vi "DSF Transfer Group.Separate Rx and Tx.vi"(8 "error in (no error)":errorcluster, 11 "Transfer Groups":refnum<class "Transfer Group.lvclass">[](array[class])) -> (0 "error out":errorcluster, 2 "Tx Transfer Groups":refnum<class "Transfer Group.lvclass">[](array[class]), 3 "Rx Transfer Groups":refnum<class "Transfer Group.lvclass">[](array[class]))   [LabVIEW 2017, in "DSF Core.lvlib" / "Transfer Group.lvclass"]
uses:
  Transfer Group.lvclass
  Transfer Group.lvclass/Transfer Group.ctl
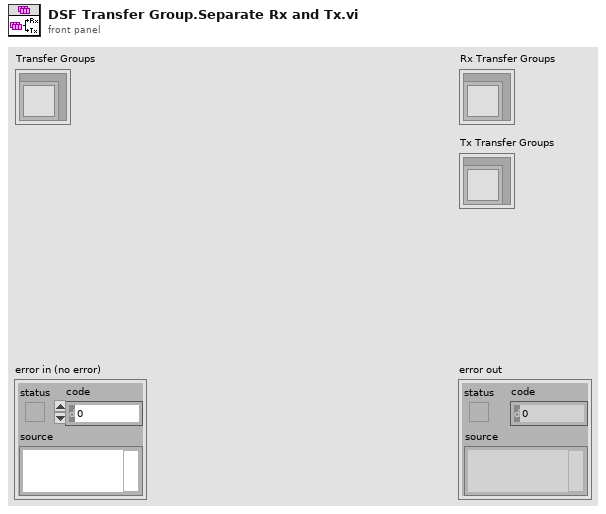
[diagram p1: front panel]
types:
  T1 = typedef "DSF Core.lvlib/DSF Direction.ctl" = enum8{"Tx", "Rx"}
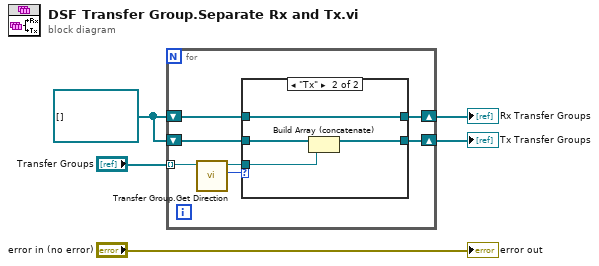
[diagram p0: block diagram]
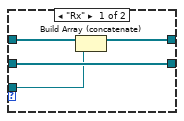
[diagram p2: hidden frame]
diagram:
  w3 = refnum<class "Transfer Group.lvclass">[] [] ("Rx Transfer Groups")
  n1 = for {
    tunnel: "Transfer Groups" -> [w10] mode=indexing
    shift-right: [w8] -> w1
    shift-left: w3 -> [w9]
    shift-right: [w6] -> w2
    shift-left: w3 -> [w7]
    n2 = call "Transfer Group.Get Direction.vi"("Transfer Group in"=w10) -> ("Direction"=w12:T1, "Transfer Group out"=w11:refnum<class "Transfer Group.lvclass">)  [unwired: 9 in]
    n3 = case shown="\"Tx\"" w12 {
      tunnel: w11 -> [w13 w20]
      tunnel: w9 -> [w14 w19]
      tunnel: [w14 w18] -> w8
      tunnel: w7 -> [w16 w17]
      tunnel: [w15 w17] -> w6
      frame "Rx" {
        n4 = Build Array (concatenate)(w16, w13) -> (w15:refnum<class "Transfer Group.lvclass">[])
      }
      frame "Tx" {
        n5 = Build Array (concatenate)(w19, w20) -> (w18:refnum<class "Transfer Group.lvclass">[])
      }
    }
  }
  "Rx Transfer Groups" <- w2
  "Tx Transfer Groups" <- w1
  "error out" <- "error in (no error)"
